vi "Initialize.vi"(8 "error in (no error)":errorcluster, 11 "WriteDigital in":refnum<class "WriteDigital.lvclass">) -> (0 "error out":errorcluster, 3 "WriteDigital out":refnum<class "WriteDigital.lvclass">)   [LabVIEW 2013, in "HardwareCharacterization.lvlib" / "WriteDigital.lvclass"]
uses:
  WriteDigital.lvclass
  Elements.ctl
  Element-XML.lvclass/Element-XML.ctl
  Write Element.vi
  Element-XML.lvclass
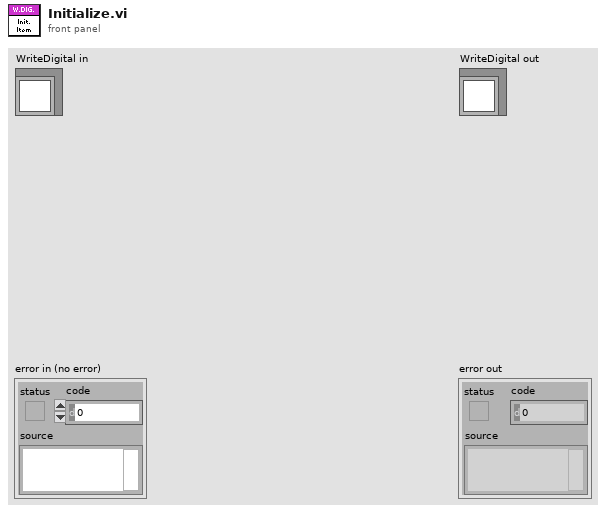
[diagram p1: front panel]
types:
  T1 = typedef "HardwareCharacterization.lvlib/Element-XML.lvclass/Elements.ctl" = enum16{"BeginJob", "WriteDigital", "WriteAnalog", "Set", "ApplicationEvent", "JumpAbs", "MarkAbs", "JumpRel", "MarkRel", "LongDelay", "EndJob"}
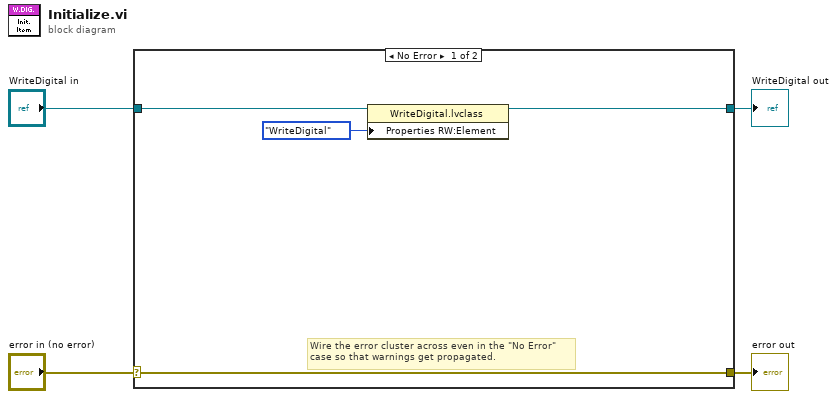
[diagram p0: block diagram]
diagram:
  n1 = case shown="No Error" "error in (no error)" {
    selector: "error in (no error)" -> [w8 w10]
    tunnel: [w8 w10] -> w3
    tunnel: [w6 w9] -> w1
    tunnel: "WriteDigital in" -> [w7 w9]
    frame No Error {
      # "Wire the error cluster across even in the \"No Error\"\ncase so that warnings get propagated."
      n2 = property class="WriteDigital.lvclass"(reference=w7, "Properties RW:Element"=Elements."WriteDigital" ("Element")) -> (reference out=w6:refnum<class "WriteDigital.lvclass">)  [unwired: 1 in, 1 out]
    }
    frame Error {
    }
  }
  "error out" <- w3
  "WriteDigital out" <- w1
